vi "Initialize Attributes.vi"(8 "error in (no error)":errorcluster, 10 "Attribute Data":variant, 11 "CS++GUIActor in":refnum<class "CS++GUIActor.lvclass">) -> (0 "error out":errorcluster, 2 "Found?":bool, 3 "CS++GUIActor out":refnum<class "CS++GUIActor.lvclass">)   [LabVIEW 2015, in "CS++GUIActor.lvlib" / "CS++GUIActor.lvclass"]
doc: "Initialize object attribute.\n\nUnique resources should be allocated elsewhere!"
uses:
  CS++GUIActor.lvclass
  CS++GUIActor.lvclass/CS++GUIActor.ctl
  CS++BaseActor/CS++BaseActor.lvclass
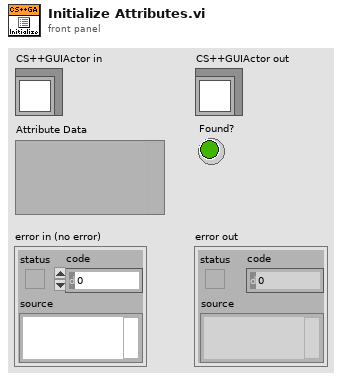
[diagram p1: front panel]
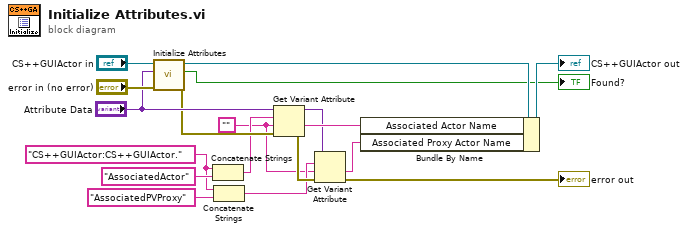
[diagram p0: block diagram]
diagram:
  w4 = ""
  w11 = "CS++GUIActor:CS++GUIActor."
  n1 = call-parent "Initialize Attributes.vi"("error in (no error)"="error in (no error)", "Attribute Data"="Attribute Data", "CS++BaseActor in"="CS++GUIActor in") -> ("error out"=w13:errorcluster, "Found?"=→"Found?":bool, "CS++BaseActor out"=w16:refnum<class "CS++GUIActor.lvclass">)  [unwired: 6 in]
  n2 = Concatenate Strings(w11, "AssociatedActor" ("string")) -> (w9:string)
  n3 = Concatenate Strings(w11, "AssociatedPVProxy" ("string")) -> (w5:string)
  n4 = Get Variant Attribute(Variant="Attribute Data", name=w9, default value (empty Variant)=w4, error in=w13) -> (duplicate Variant=w7:variant, value=w8:string, error out=w6:errorcluster)  [unwired: 1 out]
  n5 = Get Variant Attribute(Variant=w7, name=w5, default value (empty Variant)=w4, error in=w6) -> (value=w3:string, error out=→"error out":errorcluster)  [unwired: 2 out]
  n6 = Bundle By Name(cluster=w16, "Associated Actor Name"=w8, "Associated Proxy Actor Name"=w3) -> (→"CS++GUIActor out":refnum<class "CS++GUIActor.lvclass">)
